vi "sendGlobal.vi"(8 "error in (no error)":errorcluster, 10 "Function":i32, 11 "Mockbus in":refnum<class "Mockbus.lvclass">) -> (0 "error out":errorcluster, 3 "Mockbus out":refnum<class "Mockbus.lvclass">)   [LabVIEW 2015, in "Mockbus.lvclass"]
uses:
  Mockbus.lvclass
  Mockbus.lvclass/Mockbus.ctl
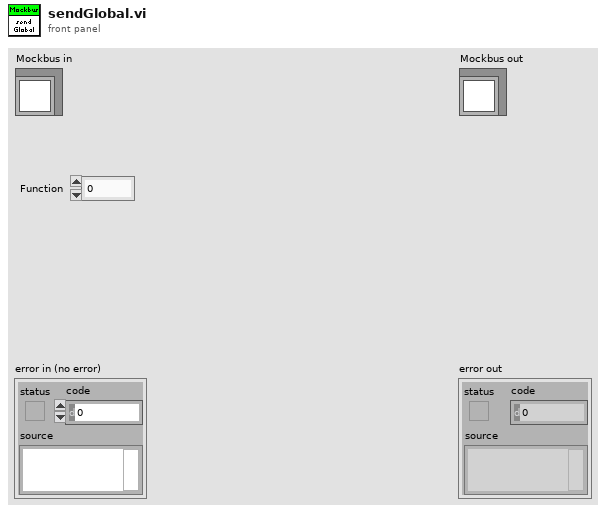
[diagram p1: front panel]
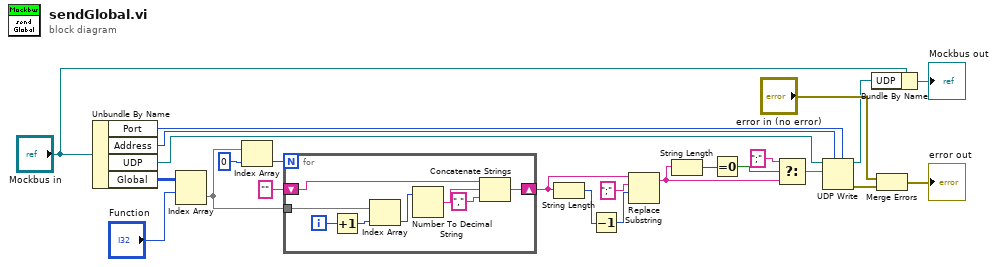
[diagram p0: block diagram]
diagram:
  n1 = Unbundle By Name("Mockbus in") -> ("Port"=w20:u16, "Address"=w21:u32, "UDP"=w22:refnum<k16>, "Global"=w23:u8[][])
  n2 = Index Array(array=w23, index (row)="Function") -> (element=w10:u8[])  [unwired: 1 in]
  n3 = Index Array(array=w10, index=0) -> (element=w11:u8)
  n4 = for {
    N: w11 -> [_]
    shift-right: [w28] -> w6
    shift-left: "" -> [w27]
    tunnel: w10 -> [w30]
    i -> [w32]
    n5 = Increment(x=w32) -> (x+1=w31:i32)
    n6 = Index Array(array=w30, index=w31) -> (element=w29:u8)
    n7 = Number To Decimal String(number=w29) -> (decimal integer string=w26:string)  [unwired: 1 in]
    n8 = Concatenate Strings(w27, w26, "," ("string")) -> (w28:string)
  }
  n9 = String Length(string=w6) -> (length=w8:i32)
  n10 = Decrement(x=w8) -> (x-1=w9:i32)
  n11 = Replace Substring(3:w9, 4:";" ("substring (\"\")"), 5:w6) -> (1:w3:string)  [unwired: 1 in, 1 out]
  n12 = String Length(string=w3) -> (length=w5:i32)
  n13 = Equal To 0?(x=w5) -> (x = 0?=w4:bool)
  n14 = Select(t=";", s=w4, f=w3) -> (s? t:f=w1:string)
  n15 = UDP Write(address=w21, port or service name=w20, connection ID=w22, data in=w1) -> (error out=w19:errorcluster, 3:w15:refnum<k16>)  [unwired: 2 in]
  n16 = Bundle By Name(cluster="Mockbus in", "UDP"=w15) -> (→"Mockbus out":refnum<class "Mockbus.lvclass">)
  n17 = Merge Errors("error in (no error)", w19) -> (→"error out":errorcluster)
